vi "Read NPin 1Sampe 1D Boolean.vi"(8 "error in (no error)":errorcluster, 10 "Pins":u8[](array[numeric]), 11 "MicroDAQ.lvlib:Digital Input.lvclass":refnum<class "Digital Input.lvclass">) -> (0 "error out":errorcluster, 2 "data":bool[](array[boolean]), 3 "MicroDAQ.lvlib:Digital Input.lvclass out":refnum<class "Digital Input.lvclass">)   [LabVIEW 2009, in "MicroDAQ.lvlib" / "Digital Input.lvclass"]
doc: "Reads a single Boolean sample from a digital input channel composed of a multiple lines."
uses:
  <instrlib>/MicroDAQ/Channel/Digital Input/Digital Input.lvclass
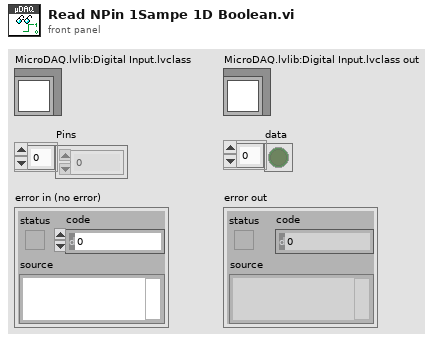
[diagram p1: front panel]
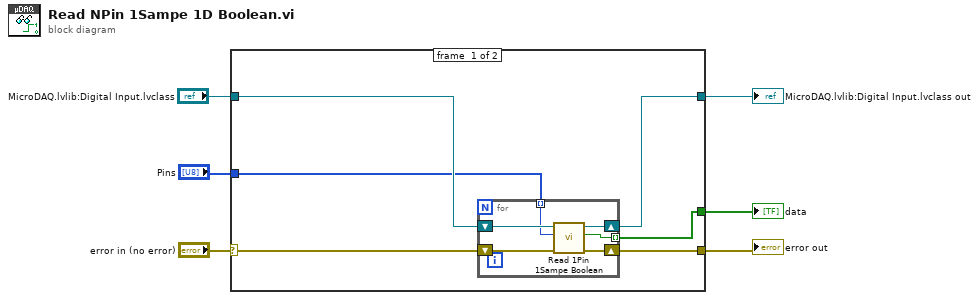
[diagram p0: block diagram]
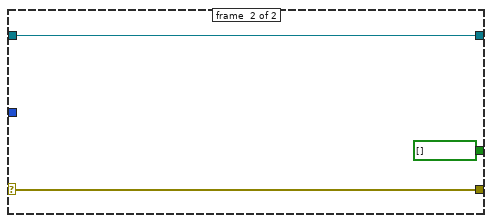
[diagram p2: hidden frame]
diagram:
  n1 = case shown="No Error" "error in (no error)" {
    selector: "error in (no error)" -> [w12 w20]
    tunnel: [w9 w20] -> w5
    tunnel: "MicroDAQ.lvlib:Digital Input.lvclass" -> [w11 w21]
    tunnel: [w10 w21] -> w3
    tunnel: "Pins" -> [w8 _]
    tunnel: [w7 bool[] []] -> w1
    frame #0 {
      n2 = for {
        shift-right: [w14] -> w9
        shift-left: w12 -> [w17]
        shift-right: [w15] -> w10
        shift-left: w11 -> [w18]
        tunnel: w8 -> [w16] mode=indexing
        tunnel: [w13] -> w7 mode=indexing
        n3 = call <instrlib>:"Read 1Pin 1Sampe Boolean.vi"("error in (no error)"=w17, "Pin"=w16, "MicroDAQ.lvlib:Digital Input.lvclass"=w18) -> ("error out"=w14:errorcluster, "data"=w13:bool, "MicroDAQ.lvlib:Digital Input.lvclass out"=w15:refnum<class "Digital Input.lvclass">)  [unwired: 6 in]
      }
    }
    frame #1 {
    }
  }
  "error out" <- w5
  "MicroDAQ.lvlib:Digital Input.lvclass out" <- w3
  "data" <- w1
